vi "XML_Header.vi"(10 "User Input":string[](array[string]), 11 "DOM document in":refnum<k20>) -> (2 "XML String Output":string, 3 "OwnerDocument":refnum<k20>)   [LabVIEW 2009]
uses:
  Program Files/National Instruments/LabVIEW 2009/resource/objmgr/DOMUserDefRef.rc
panel:
  out "appended path":path
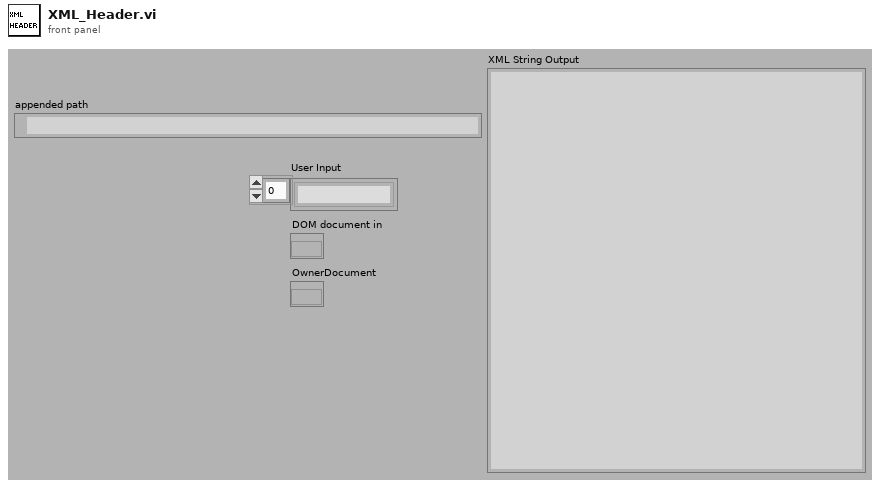
[diagram p1: front panel]
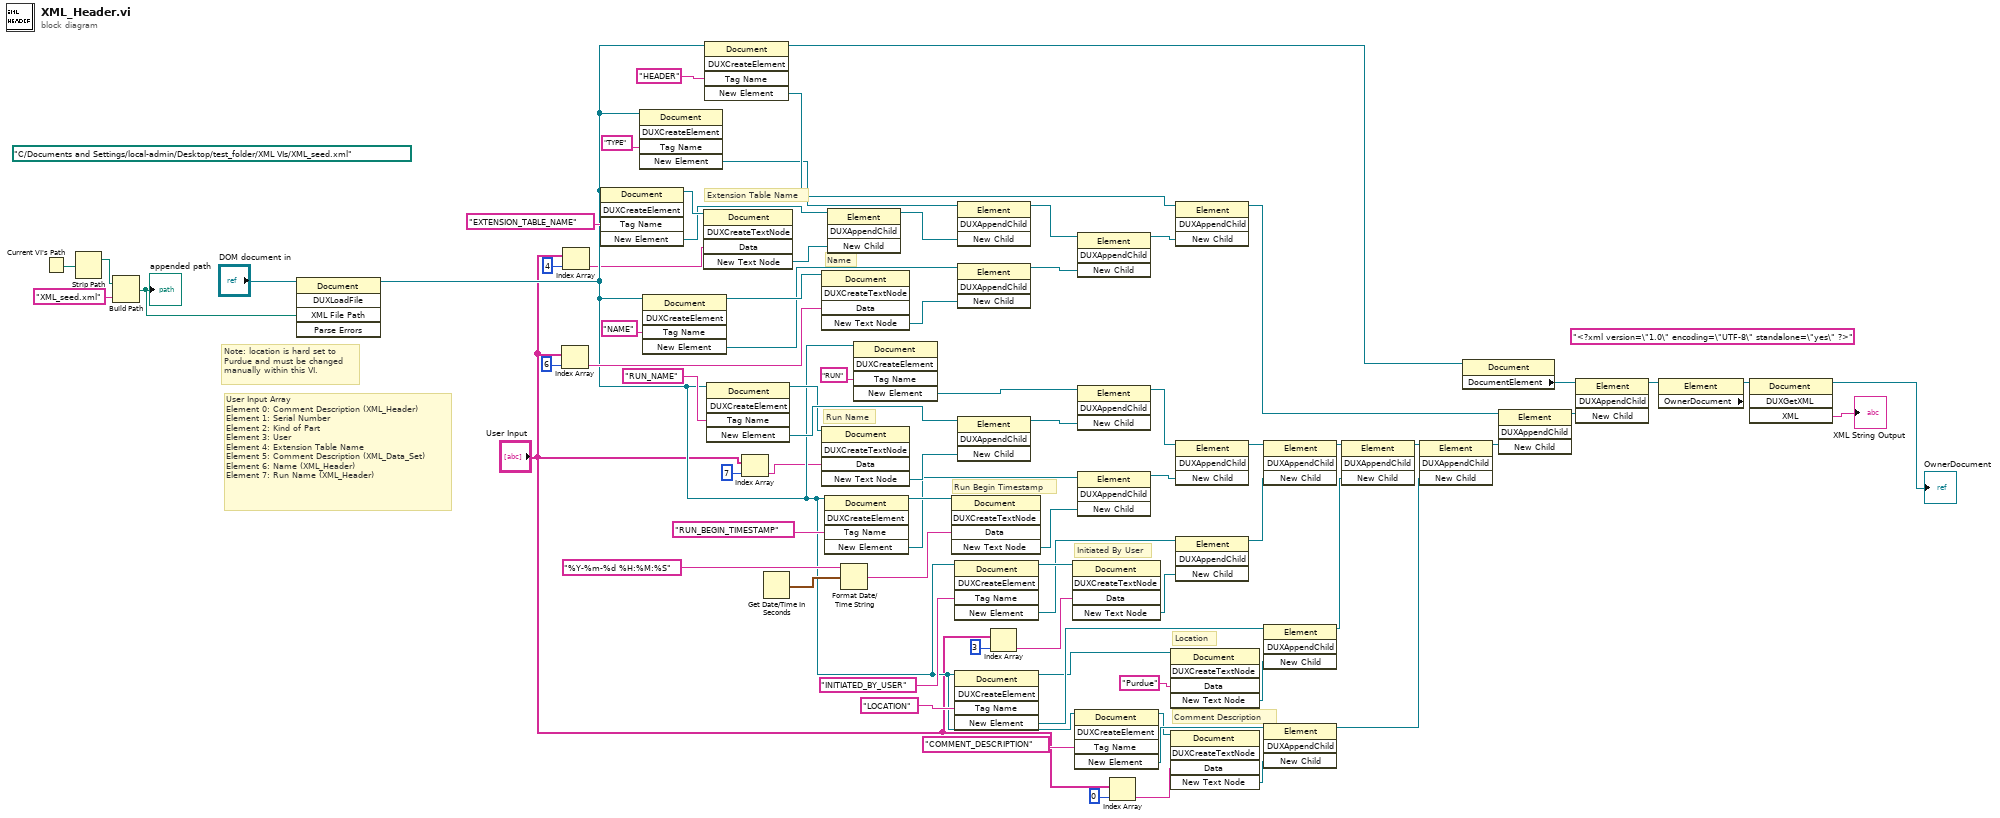
[diagram p0: block diagram]
diagram:
  (unwired) path "C:/Documents and Settings/local-admin/Desktop/test_folder/XML VIs/XML_seed.xml" ("XML File Path")
  (unwired) "<?xml version=\"1.0\" encoding=\"UTF-8\" standalone=\"yes\" ?>"
  # "User Input Array\nElement 0: Comment Description (XML_Header)\nElement 1: Serial Number\nElement 2: Kind of Part\nElement 3: User\nElement 4: Extension Table Name\nElement 5: Comment Description (XML_Data_Set)\nElement 6: Name (XML_Header)\nElement 7: Run Name (XML_Header)"
  # "Note: location is hard set to \nPurdue and must be changed\nmanually within this VI."
  # "Extension Table Name"
  # "Comment Description"
  # "Location"
  # "Initiated By User"
  # "Run Begin Timestamp"
  # "Name"
  # "Run Name"
  n1 = Current VI's Path() -> (path=w9:path)
  n2 = Strip Path(path=w9) -> (stripped path=w8:path)  [unwired: 1 out]
  n3 = Build Path(base path=w8, name or relative path="XML_seed.xml") -> (appended path=w6:path)
  "appended path" <- w6
  n4 = invoke class="Document" method="DUXLoadFile"(reference="DOM document in", "XML File Path"=w6) -> (reference out=w14:refnum<k20>)  [unwired: 3 in, 4 out]
  n5 = Index Array(array="User Input", index=6) -> (element=w26:string)
  n6 = Index Array(array="User Input", index=4) -> (element=w4:string)
  n7 = invoke class="Document" method="DUXCreateElement"(reference=w14, "Tag Name"="EXTENSION_TABLE_NAME") -> (reference out=w71:refnum<k20>, "New Element"=w69:refnum<k20>)  [unwired: 3 in, 3 out]
  n8 = invoke class="Document" method="DUXCreateElement"(reference=w14, "Tag Name"="TYPE") -> ("New Element"=w66:refnum<k20>)  [unwired: 3 in, 4 out]
  n9 = invoke class="Document" method="DUXCreateElement"(reference=w14, "Tag Name"="NAME") -> (reference out=w72:refnum<k20>, "New Element"=w70:refnum<k20>)  [unwired: 3 in, 3 out]
  n10 = invoke class="Document" method="DUXCreateTextNode"(reference=w71, "Data"=w4) -> ("New Text Node"=w73:refnum<k20>)  [unwired: 3 in, 4 out]
  n11 = invoke class="Document" method="DUXCreateElement"(reference=w14, "Tag Name"="HEADER") -> (reference out=w13:refnum<k20>, "New Element"=w67:refnum<k20>)  [unwired: 3 in, 3 out]
  n12 = invoke class="Document" method="DUXCreateElement"(reference=w14, "Tag Name"="RUN_NAME") -> (reference out=w45:refnum<k20>, "New Element"=w46:refnum<k20>)  [unwired: 3 in, 3 out]
  n13 = Index Array(array="User Input", index=7) -> (element=w2:string)
  n14 = Get Date/Time In Seconds() -> (seconds since 1Jan1904=w25:timestamp)
  n15 = invoke class="Document" method="DUXCreateTextNode"(reference=w72, "Data"=w26) -> ("New Text Node"=w74:refnum<k20>)  [unwired: 3 in, 4 out]
  n16 = invoke class="Document" method="DUXCreateTextNode"(reference=w45, "Data"=w2) -> ("New Text Node"=w47:refnum<k20>)  [unwired: 3 in, 4 out]
  n17 = invoke class="Document" method="DUXCreateElement"(reference=w14, "Tag Name"="RUN_BEGIN_TIMESTAMP") -> (reference out=w44:refnum<k20>, "New Element"=w43:refnum<k20>)  [unwired: 3 in, 3 out]
  n18 = invoke class="Element" method="DUXAppendChild"(reference=w69, "New Child"=w73) -> (reference out=w65:refnum<k20>)  [unwired: 2 in, 3 out]
  n19 = Format Date/Time String(time format string (%c)="%Y-%m-%d %H:%M:%S", seconds (now)=w25) -> (date/time string=w23:string)  [unwired: 1 in]
  n20 = invoke class="Document" method="DUXCreateElement"(reference=w14, "Tag Name"="RUN") -> ("New Element"=w29:refnum<k20>)  [unwired: 3 in, 4 out]
  n21 = invoke class="Document" method="DUXCreateTextNode"(reference=w44, "Data"=w23) -> ("New Text Node"=w48:refnum<k20>)  [unwired: 3 in, 4 out]
  n22 = invoke class="Document" method="DUXCreateElement"(reference=w14, "Tag Name"="INITIATED_BY_USER") -> (reference out=w42:refnum<k20>, "New Element"=w41:refnum<k20>)  [unwired: 3 in, 3 out]
  n23 = invoke class="Document" method="DUXCreateElement"(reference=w14, "Tag Name"="LOCATION") -> (reference out=w51:refnum<k20>, "New Element"=w52:refnum<k20>)  [unwired: 3 in, 3 out]
  n24 = invoke class="Element" method="DUXAppendChild"(reference=w66, "New Child"=w65) -> (reference out=w64:refnum<k20>)  [unwired: 2 in, 3 out]
  n25 = invoke class="Element" method="DUXAppendChild"(reference=w70, "New Child"=w74) -> (reference out=w63:refnum<k20>)  [unwired: 2 in, 3 out]
  n26 = invoke class="Element" method="DUXAppendChild"(reference=w46, "New Child"=w47) -> (reference out=w37:refnum<k20>)  [unwired: 2 in, 3 out]
  n27 = Index Array(array="User Input", index=3) -> (element=w21:string)
  n28 = invoke class="Document" method="DUXCreateTextNode"(reference=w42, "Data"=w21) -> ("New Text Node"=w49:refnum<k20>)  [unwired: 3 in, 4 out]
  n29 = invoke class="Document" method="DUXCreateElement"(reference=w14, "Tag Name"="COMMENT_DESCRIPTION") -> (reference out=w54:refnum<k20>, "New Element"=w55:refnum<k20>)  [unwired: 3 in, 3 out]
  n30 = invoke class="Element" method="DUXAppendChild"(reference=w64, "New Child"=w63) -> (reference out=w62:refnum<k20>)  [unwired: 2 in, 3 out]
  n31 = invoke class="Element" method="DUXAppendChild"(reference=w29, "New Child"=w37) -> (reference out=w40:refnum<k20>)  [unwired: 2 in, 3 out]
  n32 = invoke class="Element" method="DUXAppendChild"(reference=w43, "New Child"=w48) -> (reference out=w36:refnum<k20>)  [unwired: 2 in, 3 out]
  n33 = Index Array(array="User Input", index=0) -> (element=w19:string)
  n34 = invoke class="Document" method="DUXCreateTextNode"(reference=w51, "Data"="Purdue") -> ("New Text Node"=w50:refnum<k20>)  [unwired: 3 in, 4 out]
  n35 = invoke class="Document" method="DUXCreateTextNode"(reference=w54, "Data"=w19) -> ("New Text Node"=w53:refnum<k20>)  [unwired: 3 in, 4 out]
  n36 = invoke class="Element" method="DUXAppendChild"(reference=w67, "New Child"=w62) -> (reference out=w31:refnum<k20>)  [unwired: 2 in, 3 out]
  n37 = invoke class="Element" method="DUXAppendChild"(reference=w40, "New Child"=w36) -> (reference out=w39:refnum<k20>)  [unwired: 2 in, 3 out]
  n38 = invoke class="Element" method="DUXAppendChild"(reference=w41, "New Child"=w49) -> (reference out=w35:refnum<k20>)  [unwired: 2 in, 3 out]
  n39 = invoke class="Element" method="DUXAppendChild"(reference=w39, "New Child"=w35) -> (reference out=w38:refnum<k20>)  [unwired: 2 in, 3 out]
  n40 = invoke class="Element" method="DUXAppendChild"(reference=w52, "New Child"=w50) -> (reference out=w34:refnum<k20>)  [unwired: 2 in, 3 out]
  n41 = invoke class="Element" method="DUXAppendChild"(reference=w55, "New Child"=w53) -> (reference out=w32:refnum<k20>)  [unwired: 2 in, 3 out]
  n42 = invoke class="Element" method="DUXAppendChild"(reference=w38, "New Child"=w34) -> (reference out=w33:refnum<k20>)  [unwired: 2 in, 3 out]
  n43 = invoke class="Element" method="DUXAppendChild"(reference=w33, "New Child"=w32) -> (reference out=w30:refnum<k20>)  [unwired: 2 in, 3 out]
  n44 = property class="Document"(reference=w13) -> ("DocumentElement"=w17:refnum<k20>)  [unwired: 1 in, 2 out]
  n45 = invoke class="Element" method="DUXAppendChild"(reference=w31, "New Child"=w30) -> (reference out=w18:refnum<k20>)  [unwired: 2 in, 3 out]
  n46 = invoke class="Element" method="DUXAppendChild"(reference=w17, "New Child"=w18) -> (reference out=w15:refnum<k20>)  [unwired: 2 in, 3 out]
  n47 = property class="Element"(reference=w15) -> ("OwnerDocument"=w16:refnum<k20>)  [unwired: 1 in, 2 out]
  n48 = invoke class="Document" method="DUXGetXML"(reference=w16) -> (reference out=→"OwnerDocument":refnum<k20>, "XML"=→"XML String Output":string)  [unwired: 3 in, 2 out]
